vi "Calculate_XOR_CRC.vi"(8 "No. of Bytes for Calculation":i32, 9 "Start Position (Byte)":i32, 11 "U8 Byte Array":u8[](array[numeric])) -> (2 "CRC":u8)   [LabVIEW 2017]
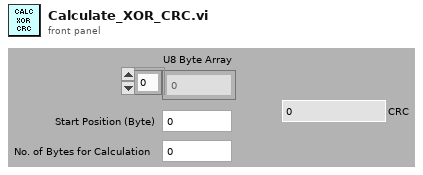
[diagram p1: front panel]
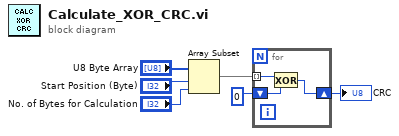
[diagram p0: block diagram]
diagram:
  n1 = Array Subset(array="U8 Byte Array", index="Start Position (Byte)", length="No. of Bytes for Calculation") -> (w5:u8[])
  n2 = for {
    shift-right: [w8] -> w4
    shift-left: u8 0 -> [w9]
    tunnel: w5 -> [w7] mode=indexing
    n3 = Exclusive Or(1:w9, 2:w7) -> (0:w8:u8)
  }
  "CRC" <- w4
